vi "Construct_Bad_Track_Except_(11-111)_Point-2.vi"(6 "[IN] Indexes for Jumps":i32[](array[numeric]), 8 "error IN":errorcluster, 9 "[IN] Index of recon\nstructed tracks":i32, 10 "[IN] Clusters for Re\nconstructed Tracks":T1, 11 "[IN] Still connected\ntracks in group":T2) -> (0 "error OUT":errorcluster, 2 "[OUT] Clusters for Re\nconstructed Tracks":T1)   [LabVIEW 2013]
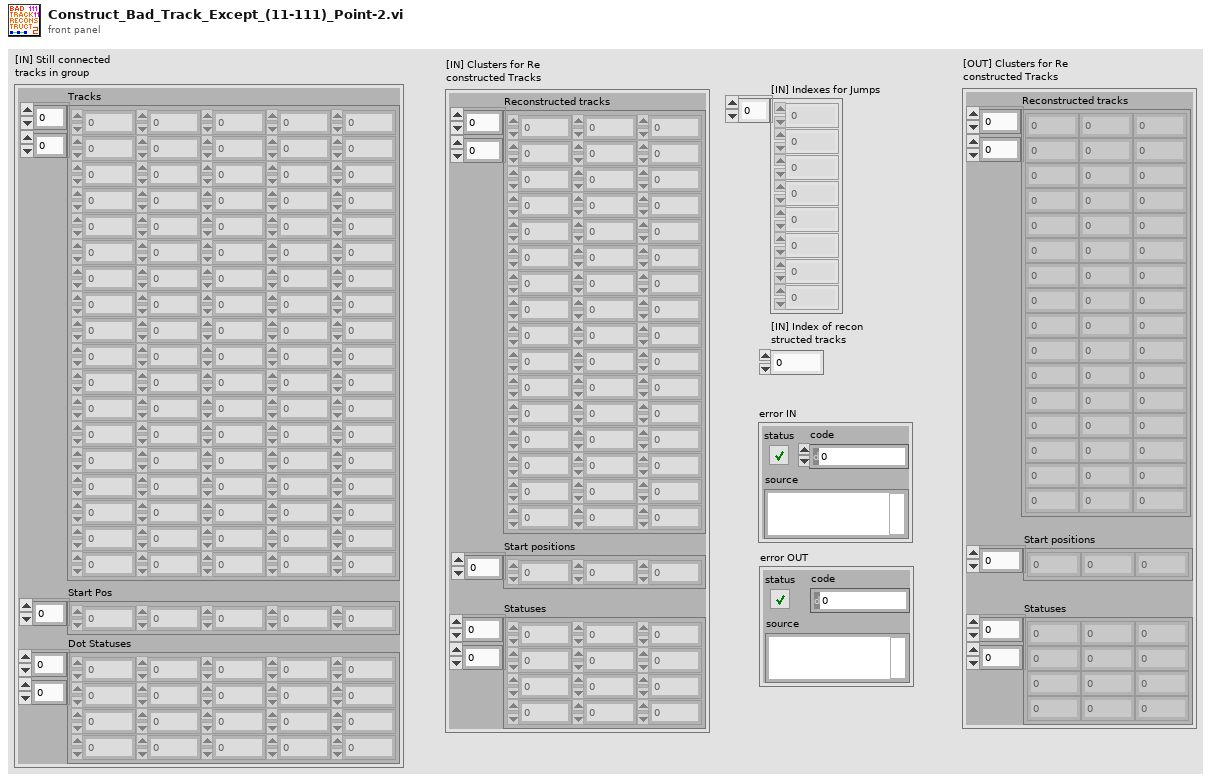
[diagram p1: front panel]
types:
  T1 = cluster{"Reconstructed tracks":dbl[][], "Start positions":i32[], "Statuses":i16[][]}
  T2 = cluster{"Tracks":dbl[][], "Start Pos":i32[], "Dot Statuses":i16[][]}
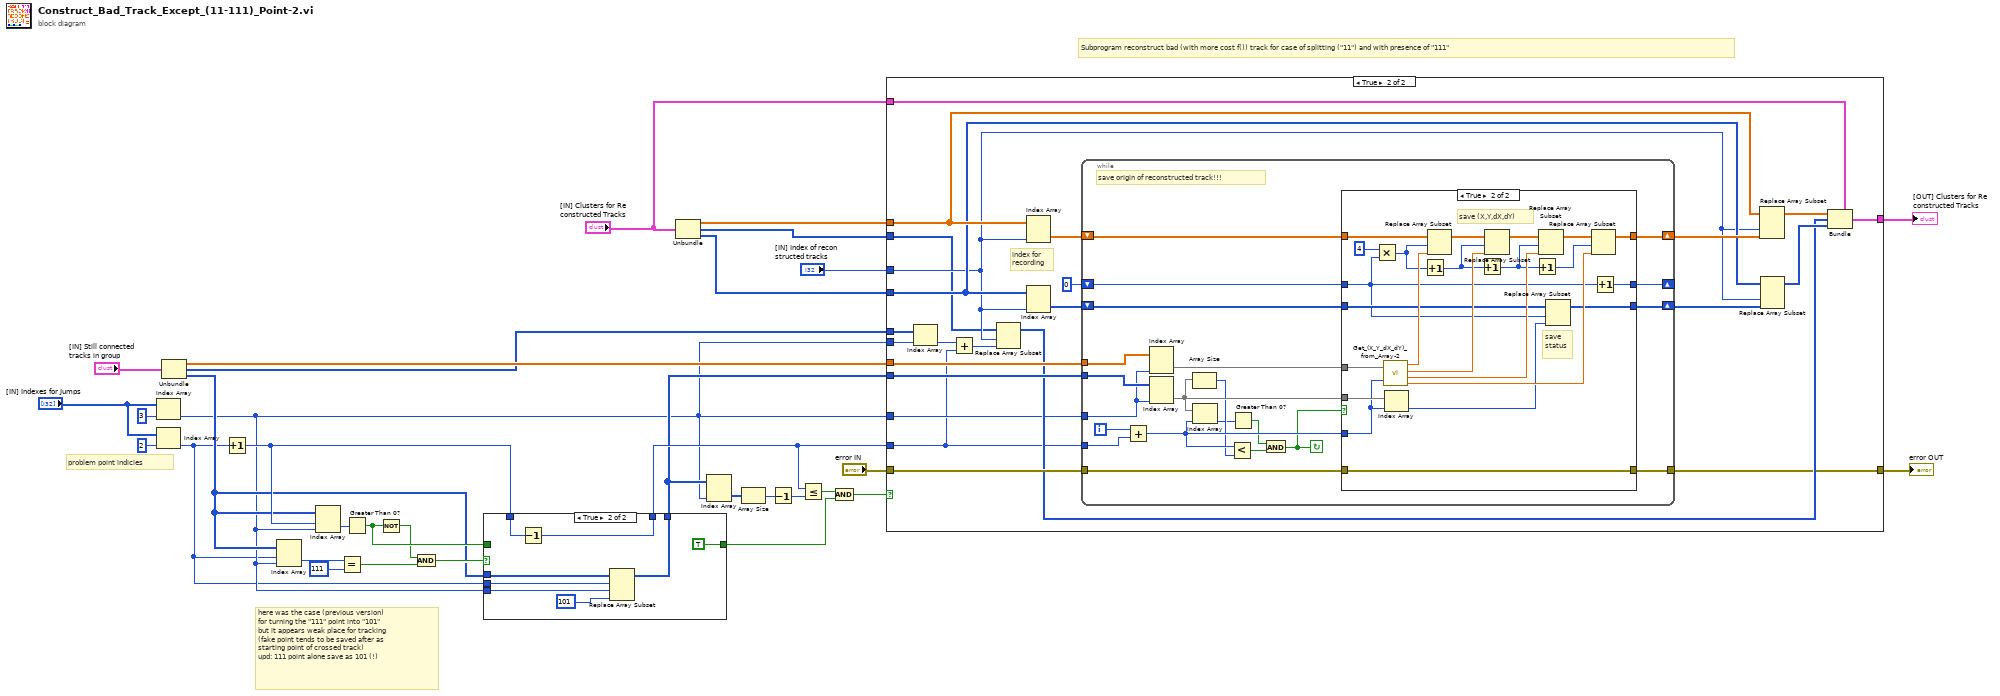
[diagram p0: block diagram]
diagram:
  # "here was the case (previous version) \nfor turning the \"111\" point into \"101\" \nbut it appears weak place for tracking \n(fake point tends to be saved after as \nstarting point of crossed track)\nupd: 111 point alone save as 101 (!)"
  # "problem point indicies"
  # "Subprogram reconstruct bad (with more cost f()) track for case of splitting (\"11\") and with presence of \"111\""
  n1 = Index Array(array="[IN] Indexes for Jumps", index=3) -> (element=w2:i32)
  n2 = Index Array(array="[IN] Indexes for Jumps", index=2) -> (element=w1:i32)
  n3 = Unbundle("[IN] Still connected\ntracks in group") -> ("Tracks"=w29:dbl[][], "Start Pos"=w15:i32[], "Dot Statuses"=w4:i16[][])
  n4 = Increment(x=w1) -> (x+1=w6:i32)
  n5 = Index Array(array=w4, index (row)=w1, index (col)=w2) -> (element=w13:i16)
  n6 = Index Array(array=w4, index (row)=w6, index (col)=w2) -> (element=w24:i16)
  n7 = Equal?(x=w13, y=i16 111) -> (x = y?=w11:bool)
  n8 = Greater Than 0?(x=w24) -> (x > 0?=w9:bool)
  n9 = Not(x=w9) -> (.not. x?=w5:bool)
  n10 = And(x=w5, y=w11) -> (x .and. y?=w10:bool)
  n11 = case shown="True" w10 {
    tunnel: w9 -> [w36 _]
    tunnel: [w36 TRUE] -> w8
    tunnel: [w35 w43] -> w7
    tunnel: w6 -> [w35 w44]
    tunnel: [w34 w37] -> w3
    tunnel: w4 -> [w34 w41]
    tunnel: w2 -> [_ w40]
    tunnel: w1 -> [_ w39]
    frame False {
    }
    frame True {
      n12 = Decrement(x=w44) -> (x-1=w43:i32)
      n13 = Replace Array Subset(array=w41, new element=i16 101 ("y"), index (row)=w39, index (col)=w40) -> (w37:i16[][])
    }
  }
  n14 = Unbundle("[IN] Clusters for Re\nconstructed Tracks") -> ("Reconstructed tracks"=w28:dbl[][], "Start positions"=w14:i32[], "Statuses"=w27:i16[][])
  n15 = Index Array(array=w3, index (col)=w2) -> (element=w23:i16[])  [unwired: 1 in]
  n16 = Array Size(array=w23) -> (size(s)=w22:i32)
  n17 = Decrement(x=w22) -> (x-1=w21:i32)
  n18 = Less Or Equal?(x=w7, y=w21) -> (x <= y?=w20:bool)
  n19 = And(x=w20, y=w8) -> (x .and. y?=w19:bool)
  n20 = case shown="True" w19 {
    tunnel: w29 -> [_ w67]
    tunnel: w28 -> [_ w60]
    tunnel: w27 -> [_ w59]
    tunnel: "[IN] Index of recon\nstructed tracks" -> [_ w54]
    tunnel: "error IN" -> [w45 w66]
    tunnel: w3 -> [_ w65]
    tunnel: "[IN] Clusters for Re\nconstructed Tracks" -> [w46 w61]
    tunnel: w15 -> [_ w55]
    tunnel: w2 -> [_ w57]
    tunnel: w7 -> [_ w49]
    tunnel: [w46 w51] -> w16
    tunnel: w2 -> [_ w50]
    tunnel: [w45 w48] -> w17
    tunnel: w14 -> [_ w47]
    frame False {
    }
    frame True {
      # "index for\nrecording"
      n21 = Index Array(array=w55, index=w57) -> (element=w56:i32)
      n22 = Add(x=w56, y=w49) -> (x+y=w53:i32)
      n23 = Replace Array Subset(array=w47, new element=w53, index=w54) -> (w52:i32[])
      n24 = Index Array(array=w60, index (col)=w54) -> (element=w70:dbl[])  [unwired: 1 in]
      n25 = Index Array(array=w59, index (col)=w54) -> (element=w69:i16[])  [unwired: 1 in]
      n26 = while {
        tunnel: w49 -> [w78]
        tunnel: w67 -> [w91]
        tunnel: w65 -> [w90]
        tunnel: w50 -> [w89]
        shift-right: [w84] -> w62
        shift-left: w70 -> [w88]
        shift-right: [w82] -> w58
        shift-left: w69 -> [w86]
        shift-right: [w83] -> _
        shift-left: 0 -> [w85]
        tunnel: w66 -> [w81]
        tunnel: [w80] -> w48
        i -> [w79]
        stop <- w71 continue-if-true
        # "save origin of reconstructed track!!!"
        n27 = Add(x=w79, y=w78) -> (x+y=w77:i32)
        n28 = Index Array(array=w91, index (col)=w89) -> (element=w87:dbl[])  [unwired: 1 in]
        n29 = Index Array(array=w90, index (col)=w89) -> (element=w76:i16[])  [unwired: 1 in]
        n30 = Array Size(array=w76) -> (size(s)=w75:i32)
        n31 = Index Array(array=w76, index=w77) -> (element=w73:i16)
        n32 = Less?(x=w77, y=w75) -> (x < y?=w72:bool)
        n33 = Greater Than 0?(x=w73) -> (x > 0?=w74:bool)
        n34 = And(x=w74, y=w72) -> (x .and. y?=w71:bool)
        n35 = case shown="True" w71 {
          tunnel: w88 -> [w95 w116]
          tunnel: w87 -> [_ w118]
          tunnel: w76 -> [_ w117]
          tunnel: w77 -> [_ w101]
          tunnel: w86 -> [w93 w103]
          tunnel: [w93 w100] -> w82
          tunnel: [w95 w99] -> w84
          tunnel: w85 -> [w94 w98]
          tunnel: [w94 w97] -> w83
          tunnel: w81 -> [w92 w96]
          tunnel: [w92 w96] -> w80
          frame False {
          }
          frame True {
            # "save (X,Y,dX,dY)"
            # "save\nstatus"
            n36 = Multiply(x=4, y=w98) -> (x*y=w112:i32)
            n37 = call "Get_(X_Y_dX_dY)_from_Array-2.vi"("(X,Y,dX,dY)"=w118, "Index of Displacement"=w101) -> ("X"=w114:dbl, "Y"=w111:dbl, "dX"=w108:dbl, "dY"=w104:dbl)
            n38 = Index Array(array=w117, index=w101) -> (element=w102:i16)
            n39 = Increment(x=w112) -> (x+1=w109:i32)
            n40 = Replace Array Subset(array=w116, new element=w114, index=w112) -> (w113:dbl[])
            n41 = Increment(x=w109) -> (x+1=w107:i32)
            n42 = Replace Array Subset(array=w113, new element=w111, index=w109) -> (w110:dbl[])
            n43 = Increment(x=w107) -> (x+1=w106:i32)
            n44 = Replace Array Subset(array=w110, new element=w108, index=w107) -> (w105:dbl[])
            n45 = Replace Array Subset(array=w103, new element=w102, index=w98) -> (w100:i16[])
            n46 = Replace Array Subset(array=w105, new element=w104, index=w106) -> (w99:dbl[])
            n47 = Increment(x=w98) -> (x+1=w97:i32)
          }
        }
      }
      n48 = Replace Array Subset(array=w60, new element=w62, index (col)=w54) -> (w63:dbl[][])  [unwired: 1 in]
      n49 = Replace Array Subset(array=w59, new element=w58, index (col)=w54) -> (w64:i16[][])  [unwired: 1 in]
      n50 = Bundle(cluster=w61, "Reconstructed tracks"=w63, "Start positions"=w52, "Statuses"=w64) -> (w51:T1)
    }
  }
  "[OUT] Clusters for Re\nconstructed Tracks" <- w16
  "error OUT" <- w17
